vi "Add.vi"(0 "reference in":refnum<class "BrowerComponent.lvclass">, 1 "BrowerComponents":refnum<class "BrowerComponent.lvclass">[](array[class]), 5 "error in (no error)":errorcluster) -> (14 "reference out":refnum<class "BrowerComponent.lvclass">, 19 "error out":errorcluster)   [LabVIEW 2015, in "BrowerComponent.lvclass"]
uses:
  BrowerComponent.lvclass
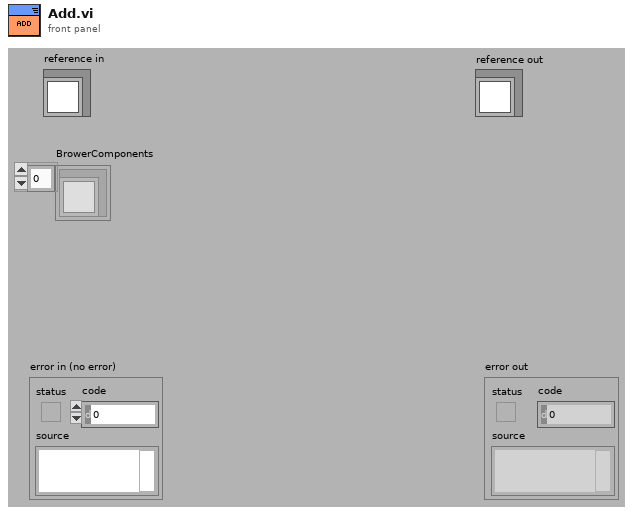
[diagram p1: front panel]
types:
  T1 = typedef "BrowerComponent.lvclass/ObjectAttributes.ctl" = cluster{"ComponentID":string, "SymbolIndex":i32, "ComponentName":string, "PartsOfComponent_dict":variant}
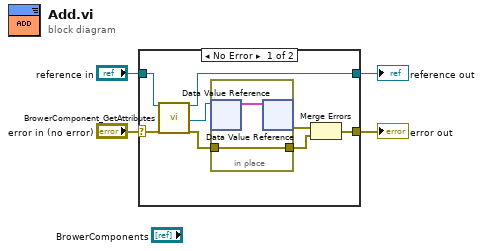
[diagram p0: block diagram]
diagram:
  n1 = case shown="No Error" "error in (no error)" {
    selector: "error in (no error)" -> [w11 w16]
    tunnel: [w8 w16] -> w3
    tunnel: [w9 w15] -> w1
    tunnel: "reference in" -> [w12 w15]
    frame No Error {
      n2 = call "BrowerComponent_GetAttributes.vi"("reference in"=w12, "error in (no error)"=w11) -> ("reference out"=w9:refnum<class "BrowerComponent.lvclass">, "DataRef"=w7:refnum<data-value>, "error out"=w6:errorcluster)  [unwired: 14 in, 1 out]
      n3 = in-place {
        in-place-border: w6 -> [w13]
        in-place-border: [w13] -> w5
        n4 = in-place-dvr #1(w7) -> (w14:T1)  [unwired: 1 out]
        n5 = in-place-dvr #1(w14) -> (w10:errorcluster)  [unwired: 1 out]
      }
      n6 = Merge Errors(w10, w5) -> (w8:errorcluster)
    }
    frame Error {
    }
  }
  "error out" <- w3
  "reference out" <- w1
